vi "Get Comm DLL Path.vi"() -> (0 "Comm DLL Path":path)   [LabVIEW 2014, in "Keyence LJ-V7000.lvlib"]
uses:
  Keyence LJ-V7000.lvlib
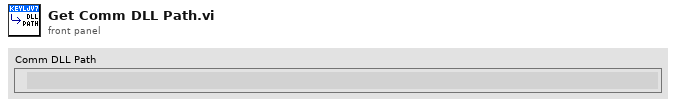
[diagram p1: front panel]
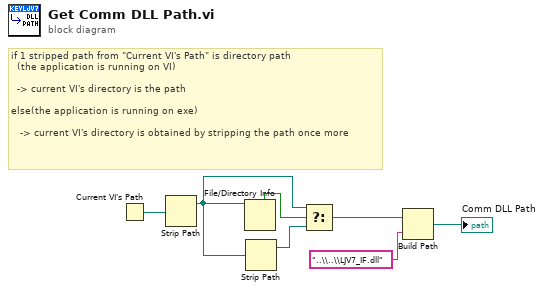
[diagram p0: block diagram]
diagram:
  # "if 1 stripped path from \"Current VI's Path\" is directory path\n  (the application is running on VI)\n\n  -> current VI's directory is the path\n\nelse(the application is running on exe)\n\n　-> current VI's directory is obtained by stripping the path once more"
  n1 = Current VI's Path() -> (path=w4:path)
  n2 = Strip Path(path=w4) -> (stripped path=w6:path)  [unwired: 1 out]
  n3 = File/Directory Info(path=w6) -> (directory=w7:bool)  [unwired: 1 in, 6 out]
  n4 = Strip Path(path=w6) -> (stripped path=w5:path)  [unwired: 1 out]
  n5 = Select(t=w6, s=w7, f=w5) -> (s? t:f=w3:path)
  n6 = Build Path(base path=w3, name or relative path="..\\..\\LJV7_IF.dll" ("名前または相対パス")) -> (appended path=→"Comm DLL Path":path)
